vi "Run All.vi"(8 "Error In":errorcluster) -> (0 "Error Out":errorcluster)   [LabVIEW 2018, in "Tests.lvlib" / "File Info.lvlib"]
uses:
  File Info.lvlib
  <vilib>/addons/_JKI Toolkits/Caraya/classes/Test/Test.lvclass
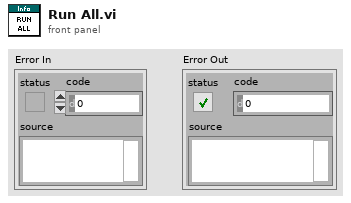
[diagram p1: front panel]
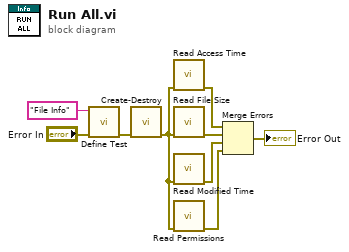
[diagram p0: block diagram]
diagram:
  n1 = call <vilib>:"Define Test.vi"("error in (no error)"="Error In", "Label (VI Title)"="File Info") -> ("error out"=w6:errorcluster)  [unwired: 9 in]
  n2 = call "Create-Destroy.vi"("Error In"=w6) -> ("Error Out"=w5:errorcluster)  [unwired: 10 in]
  n3 = call "Read Access Time.vi"("Error In"=w5) -> ("Error Out"=w4:errorcluster)  [unwired: 10 in]
  n4 = call "Read File Size.vi"("Error In"=w5) -> ("Error Out"=w3:errorcluster)  [unwired: 10 in]
  n5 = call "Read Modified Time.vi"("Error In"=w5) -> ("Error Out"=w2:errorcluster)  [unwired: 10 in]
  n6 = call "Read Permissions.vi"("Error In"=w5) -> ("Error Out"=w1:errorcluster)  [unwired: 10 in]
  n7 = Merge Errors(w4, w3, w2, w1) -> (→"Error Out":errorcluster)
